vi "SendMessageToLog.vi"(7 "Log and view ?":T1, 8 "error in (no error)":errorcluster, 10 "Message":string, 11 "Criticity":T2) -> (0 "error out":errorcluster)   [LabVIEW 2011]
uses:
  030 - EVENTS/03 - ToMessageHandlerProcess/enumMessageCriticity.ctl
  Ctrls/enumLogAndView.ctl
  030 - EVENTS/EnumFgvEventCommand.ctl
  030 - EVENTS/03 - ToMessageHandlerProcess/ToMessageHandlerEvent.ctl
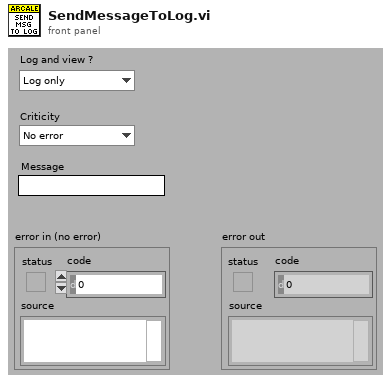
[diagram p1: front panel]
types:
  T1 = typedef "enumLogAndView.ctl" = enum16{"Log only", "Log and view"}
  T2 = typedef "enumMessageCriticity.ctl" = enum16{"No error", "Info", "Warning", "Error", "Fatal error"}
  T3 = typedef "ToMessageHandlerEvent.ctl" = cluster{"date / time":timestamp, "Criticity":T2, "Emitter":string, "Message":string}
  T4 = typedef "EnumFgvEventCommand.ctl" = enum16{"Setup", "Cleanup", "Get"}
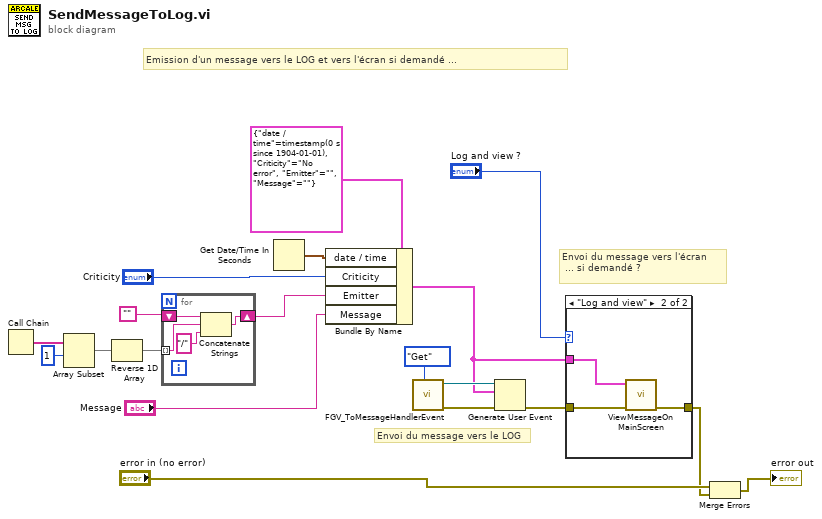
[diagram p0: block diagram]
diagram:
  # "Envoi du message vers l'écran\n ... si demandé ?"
  # "Envoi du message vers le LOG"
  # "Emission d'un message vers le LOG et vers l'écran si demandé ..."
  n1 = Call Chain() -> (call chain=w9:string[])
  n2 = Array Subset(array=w9, index=1) -> (w11:string[])  [unwired: 1 in]
  n3 = Reverse 1D Array(array=w11) -> (reversed array=w5:string[])
  n4 = for {
    tunnel: w5 -> [w21] mode=indexing
    shift-right: [w23] -> w6
    shift-left: "" -> [w22]
    n5 = Concatenate Strings(w22, w21, "/" ("string")) -> (w23:string)
  }
  n6 = Get Date/Time In Seconds() -> (seconds since 1Jan1904=w15:timestamp)
  n7 = Bundle By Name(cluster=T3 {"date / time"=timestamp(0 s since 1904-01-01), "Criticity"=enum."No error", "Emitter"="", "Message"=""} ("event data"), "date / time"=w15, "Criticity"="Criticity", "Emitter"=w6, "Message"="Message") -> (w13:T3)
  n8 = call "FGV_ToMessageHandlerEvent.vi"("Command"=EnumFgvEventCommand."Get") -> ("error out"=w18:errorcluster, "To message handler event"=w17:refnum<user-event>)  [unwired: 9 in]
  n9 = Generate User Event(user event=w17, event data cluster=w13, error in=w18) -> (error out=w14:errorcluster)  [unwired: 1 out]
  n10 = case shown="\"Log and view\"" "Log and view ?" {
    tunnel: w14 -> [w24 w27]
    tunnel: [w24 w26] -> w2
    tunnel: w13 -> [_ w25]
    frame "Log only", Default {
    }
    frame "Log and view" {
      n11 = call "ViewMessageOnMainScreen.vi"("error in (no error)"=w27, "Message"=w25) -> ("error out"=w26:errorcluster)  [unwired: 9 in]
    }
  }
  n12 = Merge Errors("error in (no error)", w2) -> (→"error out":errorcluster)
